vi "transition.vi"(8 "error in (no error)":errorcluster, 10 "ContextData In":refnum<class "ContextData.lvclass">, 11 "Run in":refnum<class "Longest.lvclass">) -> (0 "error out":errorcluster, 2 "ContextData Out":refnum<class "ContextData.lvclass">, 3 "Next Step":refnum<class "State.lvclass">)   [LabVIEW 2019, in "Longest.lvclass"]
uses:
  Longest.lvclass
  State/State.lvclass
  ContextData/ContextData.lvclass
  Wait Event/Wait Event.lvclass
  C:/Users/fflores/Documents/GitHub Projects/Simon/Simon Game/OOP States/State/State.lvclass
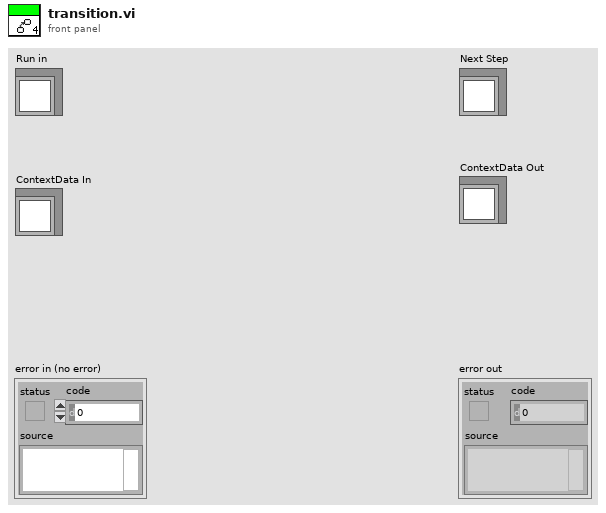
[diagram p1: front panel]
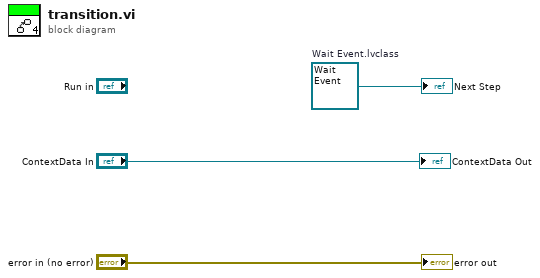
[diagram p0: block diagram]
diagram:
  w2 = refnum<class "Wait Event.lvclass"> refnum  # Wait Event.lvclass
  "error out" <- "error in (no error)"
  "Next Step" <- w2
  "ContextData Out" <- "ContextData In"
